vi "datasocket.vi"() -> ()   [LabVIEW 2011]
panel:
  out "Waveform Graph 2":dbl[](graph)
  in  "stop":bool
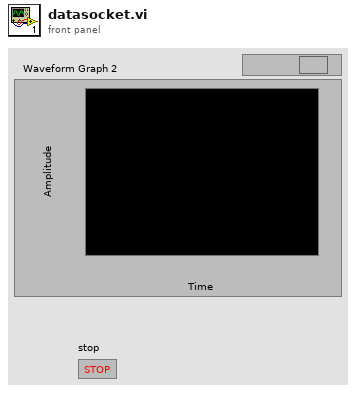
[diagram p1: front panel]
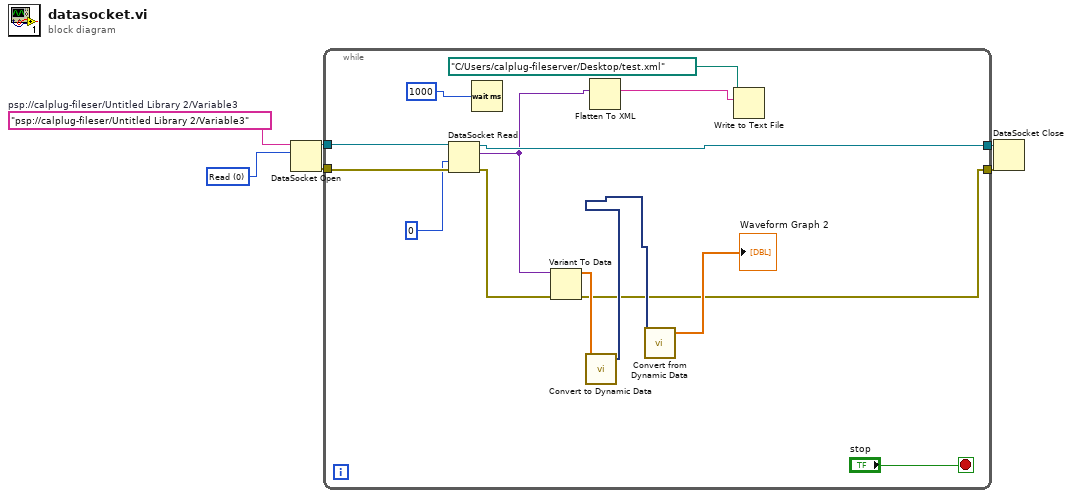
[diagram p0: block diagram]
diagram:
  w5 = u16 0 items=["Read"]
  w6 = "psp://calplug-fileser/Untitled Library 2/Variable3"  # psp://calplug-fileser/Untitled Library 2/Variable3
  n1 = DataSocket Open(10:w5, 11:w6) -> (0:w4:errorcluster, 3:w3:refnum<k13>)  [unwired: 2 in]
  n2 = while {
    tunnel: w4 -> [w17]
    tunnel: w3 -> [w18]
    tunnel: [w7] -> w2
    tunnel: [w16] -> w1
    stop <- "stop" stop-if-true
    n3 = DataSocket Read(8:w17, 9:0, 11:w18) -> (0:w8:errorcluster, 2:w12:variant, 3:w16:refnum<k13>)  [unwired: 2 in, 4 out]
    n4 = Wait (ms)(milliseconds to wait=1000) -> ()  [unwired: 1 out]
    n5 = Variant To Data(error in=w8, Variant=w12) -> (data=w10:dbl[], error out=w7:errorcluster)  [unwired: 1 in]
    n6 = call "Convert to Dynamic Data"("Array"=w10) -> ("Dynamic Data Type"=w11:dynamicdata)  [unwired: 3 in]
    n7 = Flatten To XML(anything=w12) -> (xml string=w14:string)
    n8 = call "Convert from Dynamic Data"("Dynamic Data Type"=w11) -> ("Array"=→"Waveform Graph 2":dbl[])  [unwired: 3 in]
    n9 = Write to Text File(file (use dialog)=path "C:/Users/calplug-fileserver/Desktop/test.xml", text=w14) -> ()  [unwired: 2 in, 3 out]
  }
  n10 = DataSocket Close(8:w2, 11:w1) -> ()  [unwired: 1 in, 2 out]
